vi "Database.Handler.Disconnect.vi"(6 "ReInitDLL (F)":bool, 8 "error in (no error)":errorcluster, 11 "Data in":T1) -> (0 "error out":errorcluster, 3 "Data out":T1)   [LabVIEW 2016]
doc: "Disconnect from database\n\nWabco 2017 All right reserved\nAuthor: maciej.szupienko@wabco-auto.com"
uses:
  Database.Handler.Data.ctl
  Database.Handler.Data.Status.ctl
  Database.Handler.Data.Sets.ctl
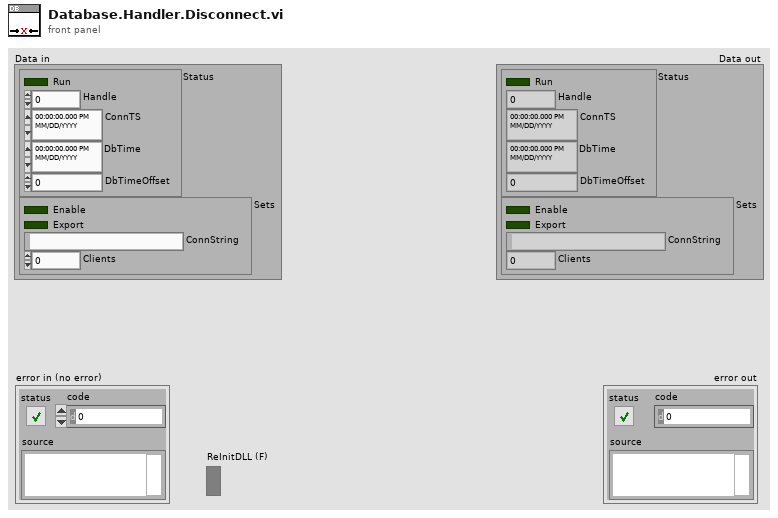
[diagram p1: front panel]
types:
  T1 = typedef "Database.Handler.Data.ctl" = cluster{"Status":T2, "Sets":T3}
  T2 = typedef "Database.Handler.Data.Status.ctl" = cluster{"Run":bool, "Handle":i32, "ConnTS":timestamp, "DbTime":timestamp, "DbTimeOffset":dbl}
  T3 = typedef "Database.Handler.Data.Sets.ctl" = cluster{"Enable":bool, "Export":bool, "ConnString":string, "Clients":i32}
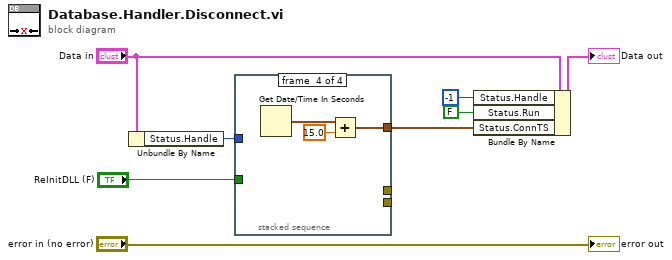
[diagram p0: block diagram]
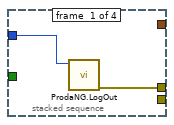
[diagram p2: hidden frame]
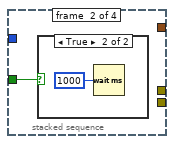
[diagram p3: hidden frame]
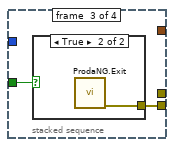
[diagram p5: hidden frame]
diagram:
  n1 = Unbundle By Name("Data in") -> ("Status.Handle"=w6:i32)
  n2 = stacked-sequence {
    tunnel: w6 -> [w10 _ _ _]
    tunnel: [w9 _ _ _] -> _
    tunnel: [_ _ _ w16] -> w3
    tunnel: [_ _ w14 _] -> _
    tunnel: "ReInitDLL (F)" -> [_ w11 w13 _]
    frame #0 {
      n3 = call "ProdaNG.LogOut.vi"("dbHandleIn"=w10) -> ("error out"=w9:errorcluster)  [unwired: 10 in]
    }
    frame #1 {
      n4 = case shown="True" w11 {
        frame False {
        }
        frame True {
          n5 = Wait (ms)(milliseconds to wait=u32 1000) -> ()  [unwired: 1 out]
        }
      }
    }
    frame #2 {
      n6 = case shown="True" w13 {
        tunnel: [_ w15] -> w14
        frame False {
        }
        frame True {
          n7 = call "ProdaNG.Exit.vi"() -> ("error out"=w15:errorcluster)  [unwired: 11 in]
        }
      }
    }
    frame #3 {
      n8 = Get Date/Time In Seconds() -> (seconds since 1Jan1904=w18:timestamp)
      n9 = Add(x=w18, y=15.0) -> (x+y=w16:timestamp)
    }
  }
  n10 = Bundle By Name(cluster="Data in", "Status.Handle"=-1, "Status.Run"=FALSE ("Status.Connected"), "Status.ConnTS"=w3) -> (→"Data out":T1)
  "error out" <- "error in (no error)"
